vi "AI-Greedy.vi"(1 "Grids":i32[][](array[numeric]), 2 "Search Depth":i32) -> (0 "BestChoice":string)   [LabVIEW 2018]
doc: "AI which using greedy algorithm.\nBe aware of CPU usage."
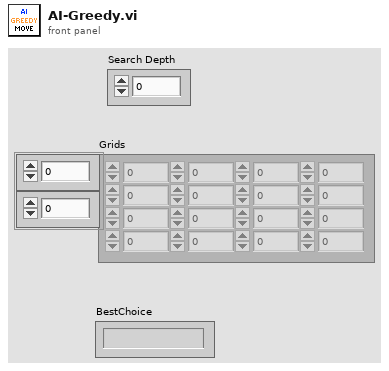
[diagram p1: front panel]
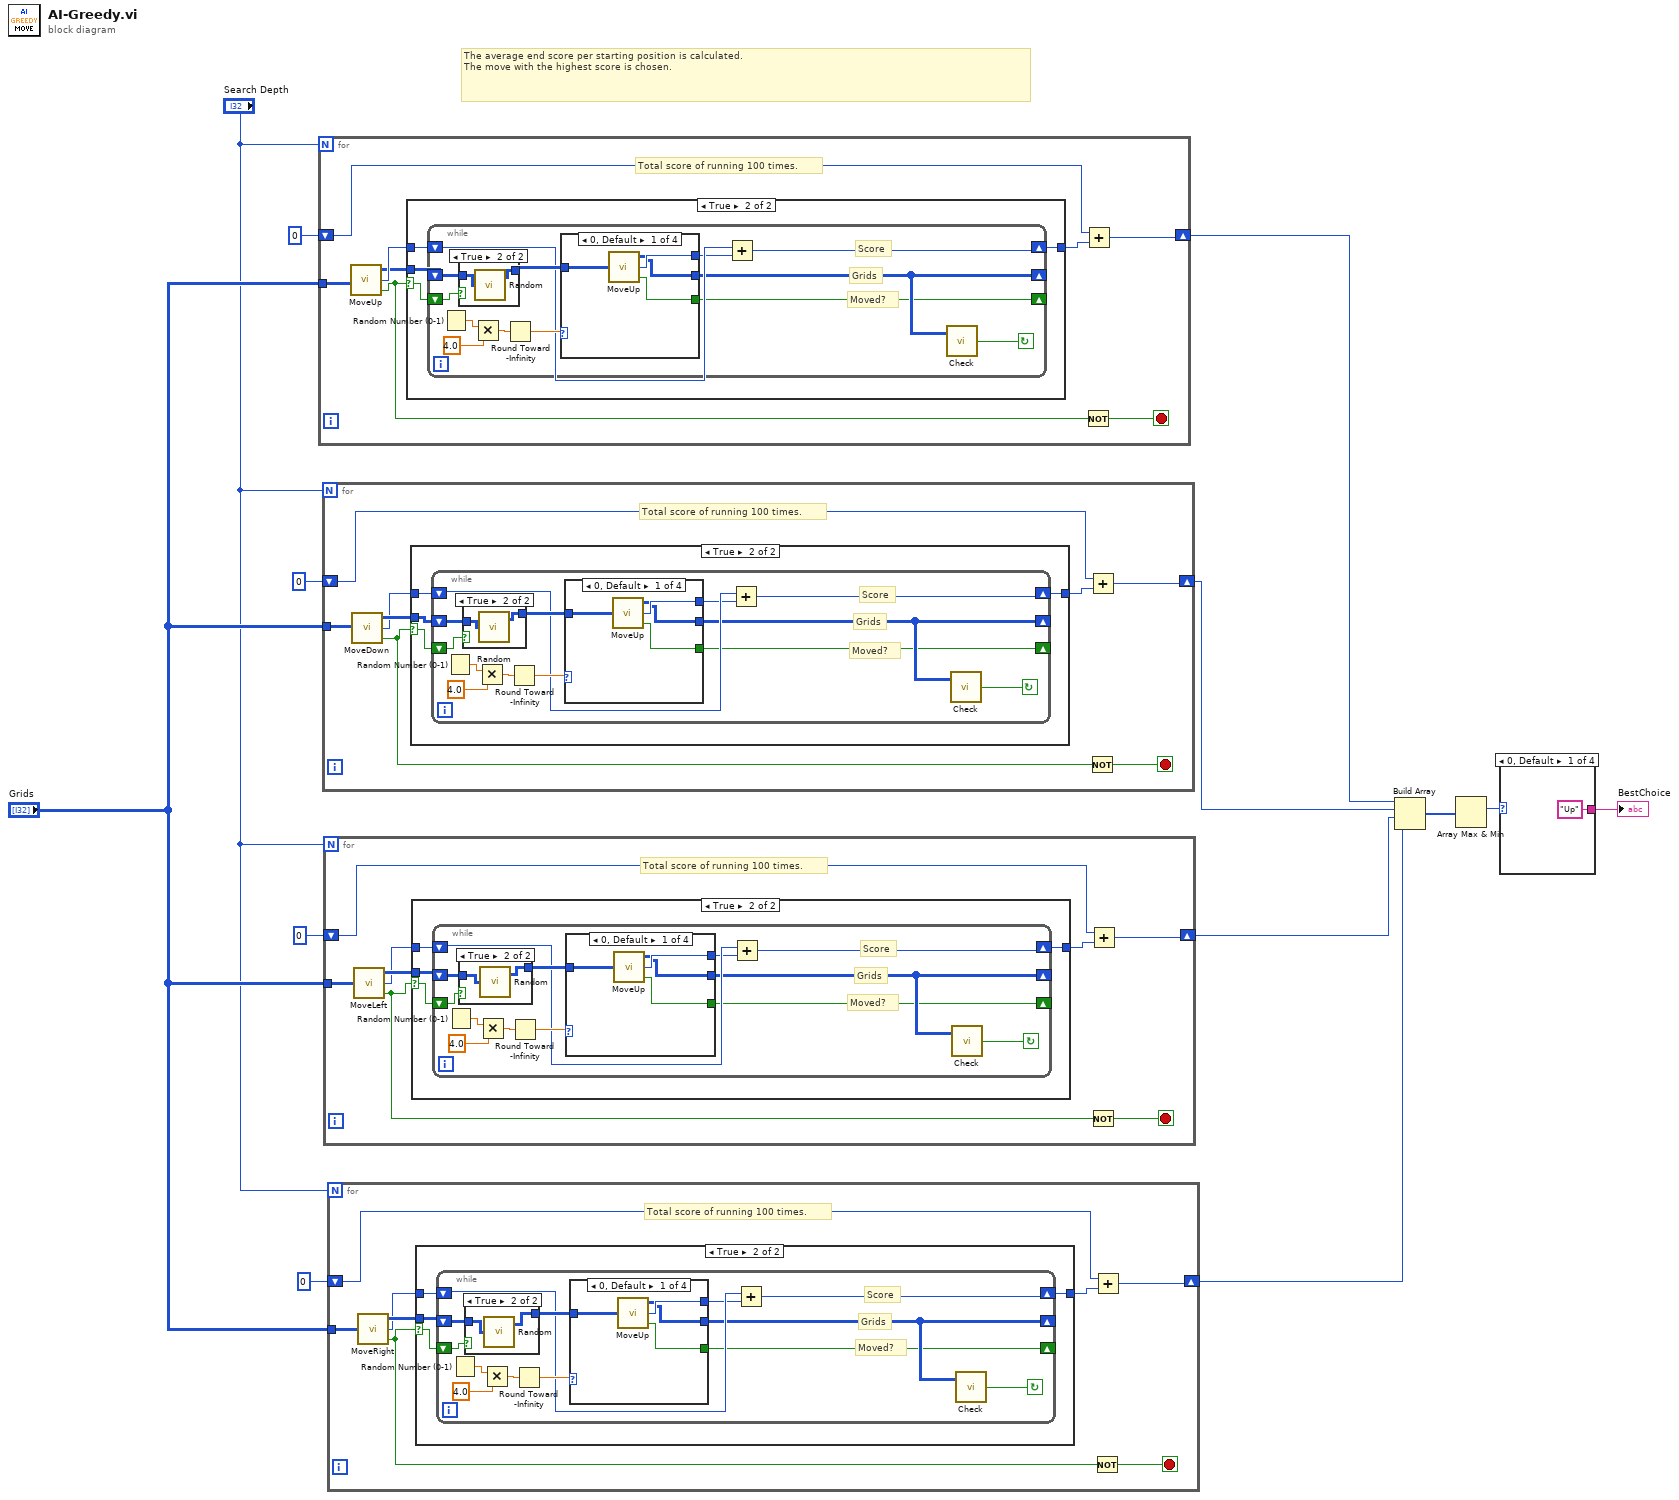
[diagram p0: block diagram]
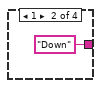
[diagram p2: hidden frame]
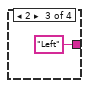
[diagram p3: hidden frame]
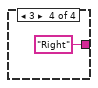
[diagram p4: hidden frame]
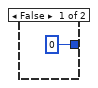
[diagram p5: hidden frame]
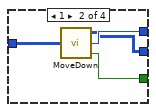
[diagram p7: hidden frame]
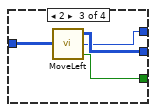
[diagram p8: hidden frame]
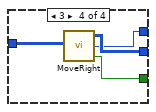
[diagram p9: hidden frame]
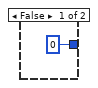
[diagram p10: hidden frame]
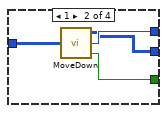
[diagram p12: hidden frame]
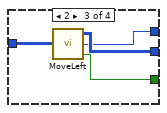
[diagram p13: hidden frame]
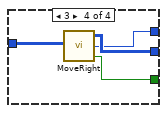
[diagram p14: hidden frame]
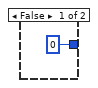
[diagram p15: hidden frame]
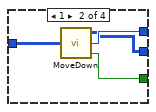
[diagram p17: hidden frame]
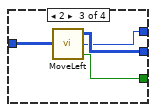
[diagram p18: hidden frame]
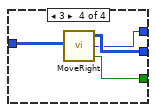
[diagram p19: hidden frame]
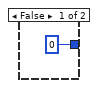
[diagram p20: hidden frame]
diagram:
  # "The average end score per starting position is calculated. \nThe move with the highest score is chosen."
  n1 = for {
    N: "Search Depth" -> [_]
    tunnel: "Grids" -> [w21]
    shift-right: [w16] -> w8
    shift-left: 0 -> [w18]
    stop <- w14 stop-if-true
    # "Total score of running 100 times."
    n2 = call "MoveUp.vi"("Grids In"=w21) -> ("Grids Out"=w19:i32[][], "Score"=w20:i32, "Moved?"=w15:bool)
    n3 = case shown="True" w15 {
      selector: w15 -> [_ w23]
      tunnel: w20 -> [_ w26]
      tunnel: w19 -> [_ w25]
      tunnel: [0 ("Score") w24] -> w17
      frame False {
      }
      frame True {
        n4 = while {
          shift-right: [w30] -> w24
          shift-left: w26 -> [w32]
          shift-right: [w29] -> _
          shift-left: w25 -> [w38]
          shift-right: [w28] -> _
          shift-left: w23 -> [w27]
          stop <- w39 continue-if-true
          # "Moved?"
          # "Grids"
          # "Score"
          n5 = Random Number (0-1)() -> (number: 0 to 1=w37:dbl)
          n6 = case shown="True" w27 {
            tunnel: w38 -> [w40 w42]
            tunnel: [w40 w41] -> w33
            frame False {
            }
            frame True {
              n7 = call "Random.vi"("Grids in"=w42) -> ("Grids out"=w41:i32[][])  [unwired: 1 out]
            }
          }
          n8 = Multiply(x=w37, y=4.0) -> (x*y=w35:dbl)
          n9 = Round Toward -Infinity(1:w35) -> (0:w34:dbl)
          n10 = case shown="0, Default" w34 {
            tunnel: w33 -> [w46 w50 w54 w58]
            tunnel: [w45 w49 w52 w56] -> w31
            tunnel: [w44 w48 w53 w57] -> w29
            tunnel: [w43 w47 w51 w55] -> w28
            frame 0, Default {
              n11 = call "MoveUp.vi"("Grids In"=w46) -> ("Grids Out"=w44:i32[][], "Score"=w45:i32, "Moved?"=w43:bool)
            }
            frame 1 {
              n12 = call "MoveDown.vi"("Grids In"=w50) -> ("Grids Out"=w48:i32[][], "Score"=w49:i32, "Moved?"=w47:bool)
            }
            frame 2 {
              n13 = call "MoveLeft.vi"("Grids In"=w54) -> ("Grid Out"=w53:i32[][], "Score"=w52:i32, "Moved?"=w51:bool)
            }
            frame 3 {
              n14 = call "MoveRight.vi"("Grids In"=w58) -> ("Grids Out"=w57:i32[][], "Score"=w56:i32, "Moved?"=w55:bool)
            }
          }
          n15 = Add(x=w32, y=w31) -> (x+y=w30:i32)
          n16 = call "Check.vi"("Grids"=w29) -> ("Movable?"=w39:bool)  [unwired: 1 in]
        }
      }
    }
    n17 = Not(x=w15) -> (.not. x?=w14:bool)
    n18 = Add(x=w18, y=w17) -> (x+y=w16:i32)
  }
  n19 = for {
    N: "Search Depth" -> [_]
    shift-right: [w64] -> w7
    shift-left: 0 -> [w66]
    tunnel: "Grids" -> [w62]
    stop <- w63 stop-if-true
    # "Total score of running 100 times."
    n20 = call "MoveDown.vi"("Grids In"=w62) -> ("Grids Out"=w61:i32[][], "Score"=w60:i32, "Moved?"=w59:bool)
    n21 = case shown="True" w59 {
      selector: w59 -> [_ w68]
      tunnel: [0 ("Score") w71] -> w65
      tunnel: w61 -> [_ w70]
      tunnel: w60 -> [_ w69]
      frame False {
      }
      frame True {
        n22 = while {
          shift-right: [w75] -> w71
          shift-left: w69 -> [w77]
          shift-right: [w74] -> _
          shift-left: w70 -> [w83]
          shift-right: [w72] -> _
          shift-left: w68 -> [w73]
          stop <- w84 continue-if-true
          # "Moved?"
          # "Grids"
          # "Score"
          n23 = Random Number (0-1)() -> (number: 0 to 1=w82:dbl)
          n24 = case shown="True" w73 {
            tunnel: w83 -> [w85 w87]
            tunnel: [w85 w86] -> w78
            frame False {
            }
            frame True {
              n25 = call "Random.vi"("Grids in"=w87) -> ("Grids out"=w86:i32[][])  [unwired: 1 out]
            }
          }
          n26 = Multiply(x=w82, y=4.0) -> (x*y=w80:dbl)
          n27 = Round Toward -Infinity(1:w80) -> (0:w79:dbl)
          n28 = case shown="0, Default" w79 {
            tunnel: w78 -> [w91 w95 w99 w103]
            tunnel: [w90 w94 w97 w101] -> w76
            tunnel: [w89 w93 w98 w102] -> w74
            tunnel: [w88 w92 w96 w100] -> w72
            frame 0, Default {
              n29 = call "MoveUp.vi"("Grids In"=w91) -> ("Grids Out"=w89:i32[][], "Score"=w90:i32, "Moved?"=w88:bool)
            }
            frame 1 {
              n30 = call "MoveDown.vi"("Grids In"=w95) -> ("Grids Out"=w93:i32[][], "Score"=w94:i32, "Moved?"=w92:bool)
            }
            frame 2 {
              n31 = call "MoveLeft.vi"("Grids In"=w99) -> ("Grid Out"=w98:i32[][], "Score"=w97:i32, "Moved?"=w96:bool)
            }
            frame 3 {
              n32 = call "MoveRight.vi"("Grids In"=w103) -> ("Grids Out"=w102:i32[][], "Score"=w101:i32, "Moved?"=w100:bool)
            }
          }
          n33 = Add(x=w77, y=w76) -> (x+y=w75:i32)
          n34 = call "Check.vi"("Grids"=w74) -> ("Movable?"=w84:bool)  [unwired: 1 in]
        }
      }
    }
    n35 = Not(x=w59) -> (.not. x?=w63:bool)
    n36 = Add(x=w66, y=w65) -> (x+y=w64:i32)
  }
  n37 = for {
    N: "Search Depth" -> [_]
    shift-right: [w109] -> w6
    shift-left: 0 -> [w111]
    tunnel: "Grids" -> [w105]
    stop <- w108 stop-if-true
    # "Total score of running 100 times."
    n38 = call "MoveLeft.vi"("Grids In"=w105) -> ("Grid Out"=w107:i32[][], "Score"=w106:i32, "Moved?"=w104:bool)
    n39 = case shown="True" w104 {
      selector: w104 -> [_ w113]
      tunnel: [0 ("Score") w116] -> w110
      tunnel: w107 -> [_ w115]
      tunnel: w106 -> [_ w114]
      frame False {
      }
      frame True {
        n40 = while {
          shift-right: [w120] -> w116
          shift-left: w114 -> [w122]
          shift-right: [w119] -> _
          shift-left: w115 -> [w128]
          shift-right: [w118] -> _
          shift-left: w113 -> [w117]
          stop <- w129 continue-if-true
          # "Moved?"
          # "Grids"
          # "Score"
          n41 = Random Number (0-1)() -> (number: 0 to 1=w127:dbl)
          n42 = case shown="True" w117 {
            tunnel: w128 -> [w130 w132]
            tunnel: [w130 w131] -> w123
            frame False {
            }
            frame True {
              n43 = call "Random.vi"("Grids in"=w132) -> ("Grids out"=w131:i32[][])  [unwired: 1 out]
            }
          }
          n44 = Multiply(x=w127, y=4.0) -> (x*y=w125:dbl)
          n45 = Round Toward -Infinity(1:w125) -> (0:w124:dbl)
          n46 = case shown="0, Default" w124 {
            tunnel: w123 -> [w136 w140 w144 w148]
            tunnel: [w135 w139 w142 w146] -> w121
            tunnel: [w134 w138 w143 w147] -> w119
            tunnel: [w133 w137 w141 w145] -> w118
            frame 0, Default {
              n47 = call "MoveUp.vi"("Grids In"=w136) -> ("Grids Out"=w134:i32[][], "Score"=w135:i32, "Moved?"=w133:bool)
            }
            frame 1 {
              n48 = call "MoveDown.vi"("Grids In"=w140) -> ("Grids Out"=w138:i32[][], "Score"=w139:i32, "Moved?"=w137:bool)
            }
            frame 2 {
              n49 = call "MoveLeft.vi"("Grids In"=w144) -> ("Grid Out"=w143:i32[][], "Score"=w142:i32, "Moved?"=w141:bool)
            }
            frame 3 {
              n50 = call "MoveRight.vi"("Grids In"=w148) -> ("Grids Out"=w147:i32[][], "Score"=w146:i32, "Moved?"=w145:bool)
            }
          }
          n51 = Add(x=w122, y=w121) -> (x+y=w120:i32)
          n52 = call "Check.vi"("Grids"=w119) -> ("Movable?"=w129:bool)  [unwired: 1 in]
        }
      }
    }
    n53 = Not(x=w104) -> (.not. x?=w108:bool)
    n54 = Add(x=w111, y=w110) -> (x+y=w109:i32)
  }
  n55 = for {
    N: "Search Depth" -> [_]
    shift-right: [w154] -> w5
    shift-left: 0 -> [w156]
    tunnel: "Grids" -> [w149]
    stop <- w153 stop-if-true
    # "Total score of running 100 times."
    n56 = call "MoveRight.vi"("Grids In"=w149) -> ("Grids Out"=w152:i32[][], "Score"=w150:i32, "Moved?"=w151:bool)
    n57 = case shown="True" w151 {
      selector: w151 -> [_ w158]
      tunnel: [0 ("Score") w161] -> w155
      tunnel: w152 -> [_ w160]
      tunnel: w150 -> [_ w159]
      frame False {
      }
      frame True {
        n58 = while {
          shift-right: [w165] -> w161
          shift-left: w159 -> [w167]
          shift-right: [w164] -> _
          shift-left: w160 -> [w173]
          shift-right: [w163] -> _
          shift-left: w158 -> [w162]
          stop <- w174 continue-if-true
          # "Moved?"
          # "Grids"
          # "Score"
          n59 = Random Number (0-1)() -> (number: 0 to 1=w172:dbl)
          n60 = case shown="True" w162 {
            tunnel: w173 -> [w175 w177]
            tunnel: [w175 w176] -> w168
            frame False {
            }
            frame True {
              n61 = call "Random.vi"("Grids in"=w177) -> ("Grids out"=w176:i32[][])  [unwired: 1 out]
            }
          }
          n62 = Multiply(x=w172, y=4.0) -> (x*y=w170:dbl)
          n63 = Round Toward -Infinity(1:w170) -> (0:w169:dbl)
          n64 = case shown="0, Default" w169 {
            tunnel: w168 -> [w181 w185 w189 w193]
            tunnel: [w180 w184 w187 w191] -> w166
            tunnel: [w179 w183 w188 w192] -> w164
            tunnel: [w178 w182 w186 w190] -> w163
            frame 0, Default {
              n65 = call "MoveUp.vi"("Grids In"=w181) -> ("Grids Out"=w179:i32[][], "Score"=w180:i32, "Moved?"=w178:bool)
            }
            frame 1 {
              n66 = call "MoveDown.vi"("Grids In"=w185) -> ("Grids Out"=w183:i32[][], "Score"=w184:i32, "Moved?"=w182:bool)
            }
            frame 2 {
              n67 = call "MoveLeft.vi"("Grids In"=w189) -> ("Grid Out"=w188:i32[][], "Score"=w187:i32, "Moved?"=w186:bool)
            }
            frame 3 {
              n68 = call "MoveRight.vi"("Grids In"=w193) -> ("Grids Out"=w192:i32[][], "Score"=w191:i32, "Moved?"=w190:bool)
            }
          }
          n69 = Add(x=w167, y=w166) -> (x+y=w165:i32)
          n70 = call "Check.vi"("Grids"=w164) -> ("Movable?"=w174:bool)  [unwired: 1 in]
        }
      }
    }
    n71 = Not(x=w151) -> (.not. x?=w153:bool)
    n72 = Add(x=w156, y=w155) -> (x+y=w154:i32)
  }
  n73 = Build Array(w8, w7, w6, w5) -> (w4:i32[])
  n74 = Array Max & Min(array=w4) -> (max index (indices)=w3:i32)  [unwired: 3 out]
  n75 = case shown="0, Default" w3 {
    tunnel: ["Up" ("BestChoice") "Down" ("BestChoice") "Left" ("BestChoice") "Right" ("BestChoice")] -> w2
    frame 0, Default {
    }
    frame 1 {
    }
    frame 2 {
    }
    frame 3 {
    }
  }
  "BestChoice" <- w2
